vi "Calc Slopes.vi"(10 "side points":i32, 11 "Filtered X in":dbl[](array[numeric])) -> (1 "slopes":dbl[](array[numeric]), 2 "filtered indices":i32[](array[numeric]), 3 "filtered values":dbl[](array[numeric]), 4 "Filtered Slopes":dbl[](array[numeric]))   [LabVIEW 2017]
uses:
  <vilib>/Analysis/3filter.llb/Savitzky-Golay Filter (DBL).vi
  <vilib>/Analysis/NI_AALBase.lvlib
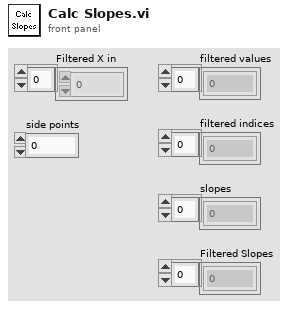
[diagram p1: front panel]
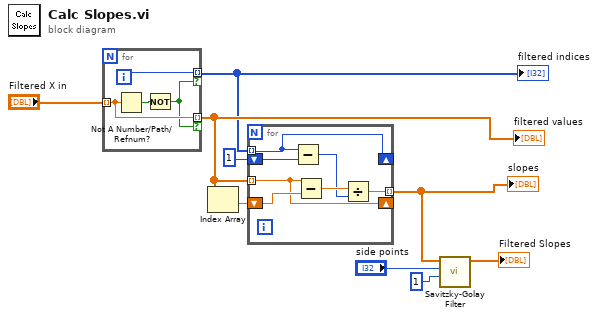
[diagram p0: block diagram]
diagram:
  n1 = for {
    tunnel: "Filtered X in" -> [w12] mode=indexing
    tunnel: [w10] -> w4 mode=indexing if=w11
    tunnel: [w12] -> w5 mode=indexing if=w11
    i -> [w10]
    n2 = Not A Number/Path/Refnum?(number/path/refnum=w12) -> (NaN/Path/Refnum?=w13:bool)
    n3 = Not(x=w13) -> (.not. x?=w11:bool)
  }
  "filtered values" <- w5
  "filtered indices" <- w4
  n4 = Index Array(array=w5) -> (element=w2:dbl)  [unwired: 1 in]
  n5 = for {
    tunnel: w5 -> [w19] mode=indexing
    shift-right: [w19] -> _
    shift-left: w2 -> [w20]
    tunnel: w4 -> [w17] mode=indexing
    shift-right: [w17] -> _
    shift-left: 1 ("index (row)") -> [w16]
    tunnel: [w15] -> w6 mode=indexing
    n6 = Subtract(x=w17, y=w16) -> (x-y=w14:i32)
    n7 = Subtract(x=w19, y=w20) -> (x-y=w18:dbl)
    n8 = Divide(x=w18, y=w14) -> (x/y=w15:dbl)
  }
  "slopes" <- w6
  n9 = call-poly <vilib>:"Savitzky-Golay Filter.vi"("polynomial order"=1, "side points"="side points", "X"=w6) -> ("Filtered X"=→"Filtered Slopes":dbl[])  [unwired: 7 in, 1 out]
